vi "Handle Command.vi"(8 "error in (no error)":errorcluster, 9 "Data":variant, 10 "Command":string, 11 "Instrument.Lockin":refnum<class "Instrument.Lockin.lvclass">) -> (0 "error out":errorcluster, 1 "Processed Data":variant, 2 "Command":string, 3 "Instrument.Lockin out":refnum<class "Instrument.Lockin.lvclass">)   [LabVIEW 2019, in "Instrument.Lockin.lvlib" / "Instrument.Lockin.lvclass"]
uses:
  Instrument.Lockin.lvclass
  Typedefs/API/Lockin.Commands--Enum.ctl
  f7b28b50-f868-4d06-8d90-790d331e6843.vi
  Instrument.DAQ/Instrument.DAQ.lvclass
  Instrument.DAQ/Typedefs/AO.Channel.Function--Enum.ctl
  Instrument.DAQ/Typedefs/AO.Channel--Cluster.ctl
  06f5bff1-b823-416c-a758-fc672ecfcc99.vi
  Typedefs/API/Lockin.setAO_Amp--cluster.ctl
  029a7bc4-99e9-4f65-b437-c26585c9cd40.vi
  95117756-58c8-4cf5-b4a1-eea4f9571e2f.vi
  d527b0ad-2cbe-40d7-81d2-49d8d0078832.vi
  c6561379-f98d-4793-93aa-fc4f7b6fa2da.vi
  Typedefs/API/Lockin.setAO_DC--cluster.ctl
  Typedefs/API/Lockin.setAO_f--cluster.ctl
  Typedefs/API/Lockin.setAO_phi--cluster.ctl
  Typedefs/API/Lockin.setAO_function--cluster.ctl
  2465c698-e437-4a4f-8860-a626a4e5f6de.vi
  3b890341-4124-4342-9d75-403cba162ea7.vi
  efd52b93-d691-4a9b-b54f-f4c6778ec2a4.vi
  1b48001d-6f4c-40ce-9883-2cfdfc5b0066.vi
  451a16e7-7f0f-4872-98b2-f896a68061ac.vi
  Instrument.DAQ/Typedefs/REF.Channel--Cluster.ctl
  Typedefs/REF Parameter--Enum.ctl
  Typedefs/API/Lockin.setREF_f--cluster.ctl
  Typedefs/API/Lockin.setREF_phi--cluster.ctl
  Typedefs/API/Lockin.setREF_TC--cluster.ctl
  Typedefs/API/Lockin.setREF_RollOff--cluster.ctl
  Instrument.DAQ/Typedefs/State--enum.ctl
  afc408c1-4a47-494c-817e-7b9f9bb33729.vi
  Instrument.DAQ/Typedefs/Sweep.Pattern--Enum.ctl
  Instrument.DAQ/Typedefs/Sweep.Channel--Cluster.ctl
  Instrument.DAQ/Typedefs/Sweep.Configuration--Cluster.ctl
  ce862ac6-3818-4682-989c-38fcf43d7c0a.vi
  06811b67-d74b-4972-af3b-9250fa170671.vi
  Instrument.DAQ/Typedefs/DAQ.Sampling.Sampling--Cluster.ctl
  2eef0b96-7480-46b2-a416-598848f5f946.vi
  b666889e-e9d3-40fa-bff7-b740bef29075.vi
  Instrument.DAQ/Typedefs/DAQ.Config.AI.Coupling--enum.ctl
  Instrument.DAQ/Typedefs/DAQ.Config.AI.Range--enum.ctl
  Instrument.DAQ/Typedefs/DAQ.Config.AO.Range--enum.ctl
  Instrument.DAQ/Typedefs/DAQ.Configuration--Cluster.ctl
  4baefe16-dd55-4900-a34f-f85402a43af0.vi
  Instrument.DAQ/Typedefs/Sweep.Channel--Cluster--Array.ctl
  Instrument.DAQ/Typedefs/AO.Channel--Cluster--Array.ctl
  Instrument.DAQ/Typedefs/REF.Channel--Cluster--Array.ctl
  Instrument.DAQ/Typedefs/DAQ.Configuration--Cluster--Array.ctl
  df248ea2-cdbc-4a64-a66c-167358fcc18f.vi
  Instrument.DAQ/Typedefs/AI.Channel--Cluster.ctl
  Instrument.DAQ/Typedefs/AI.Channel--Cluster--Array.ctl
  Typedefs/Offset Mode--Enum.ctl
  Instrument.DAQ/Typedefs/Configuration.Prefilter--Cluster.ctl
  Typedefs/API/Lockin.Commands.Local--Enum.ctl
  Instrument.DAQ/Typedefs/Configuration.LinkFrequencies--Cluster.ctl
  Instrument.DAQ/Typedefs/Configuration.AmplitudeLimit--Cluster.ctl
  Instrument.DAQ/Typedefs/Simulation Mode--enum.ctl
  Instrument.DAQ/Typedefs/Channel.Gain--Cluster.ctl
  Instrument.DAQ/Typedefs/PrivateEvents--DAQ.setCalibration.ctl
  f4b2f717-a3e3-4701-aa1a-36f1ad587562.vi
  cb03029c-6dea-422e-9ff0-c01ba24202a7.vi
  ea7ae40a-427f-4df9-8330-54c2df2a5be0.vi
  d5077292-e533-4b52-a4d7-ebb5f6280e78.vi
  be7fa38f-04e0-4644-9c08-a6c1d8484273.vi
  228c5f99-5a8a-4ac9-8c3f-6c80f04cbb43.vi
  847e6f07-fde4-45b3-9907-c341240c9864.vi
  bf5afc16-6b2f-47bd-9035-54b404507785.vi
  Instrument.DAQ/Typedefs/PrivateEvents--DAQ.showUI.ctl
  Typedefs/API/Lockin.setState--cluster.ctl
  0f1e83ab-c55c-46b9-bca3-9d617c6a026d.vi
  Typedefs/API/Lockin.setSweep_Time--cluster.ctl
  c46d61d8-ad78-4a4f-bd83-bba7d42c3393.vi
  Typedefs/API/Lockin.setSweep_Table--cluster.ctl
  <userlib>/LevyLab/Instrument Framework/Instrument Types/Lockin/Instrument.LockinAPI.lvclass
  a7ccf487-04bf-437f-bc58-012293c091eb.vi
  Typedefs/API/Lockin.setLogMode--cluster.ctl
  7fa0c9c7-d96f-42eb-b083-8fec20da1e25.vi
  <userlib>/LevyLab/Instrument Framework/Instrument Types/Lockin/Typedefs/LockinAPI.SweepData--Cluster.ctl
  <userlib>/LevyLab/Instrument Framework/Instrument Types/Lockin/Typedefs/LockinAPI.Sampling.Sampling--Cluster.ctl
  <userlib>/LevyLab/Instrument Framework/Instrument Types/Lockin/Typedefs/LockinAPI.getState.states--enum.ctl
  29174cef-b5b4-4b3d-8dd9-d067235044c7.vi
  Instrument.DAQ/Typedefs/Configuration.DCLimit--Cluster.ctl
  Instrument.DAQ/Typedefs/DAQ.TerminalConfiguration--ring.ctl
  0557ee3d-f7cd-4618-85ce-94304b7e905c.vi
  Instrument.DAQ/Typedefs/Configuration.DutyCycle--Cluster.ctl
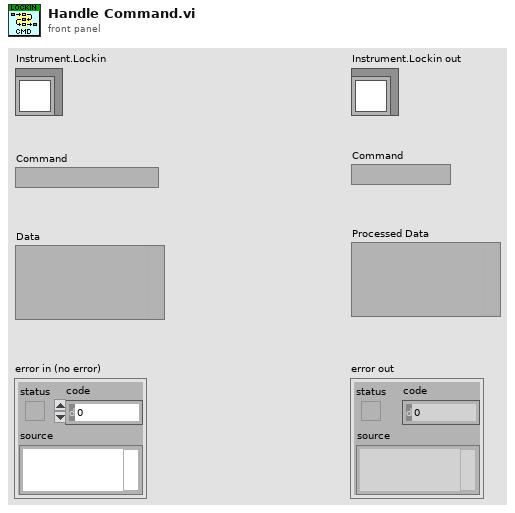
[diagram p1: front panel]
types:
  T1 = typedef "Instrument.Lockin.lvlib/Instrument.Lockin.lvclass/Lockin.Commands.Local--Enum.ctl" = enum16{"autoConfigureDAQ", "setSimulationMode", "zeroPhase", "setCalibration", "setPreFilter", "setFrequencyLink", "setAmplitudeLimit", "setDCLimit", "setDutyCycle", "setSamplingFsOutput", "setData_State", "setData_DAQ", "setData_Sampling", "setData_Waveforms", "setData_Results", "setData_SweepWaveforms", "setData_AIChannels", "setData_AOChannels", "setData_REFChannels", "setData_InputGain", "setData_OutputGain", "showUI", "setAI", "setOffset", "setOffsetMode"}
  T2 = typedef "Instrument.Lockin.lvlib/Instrument.Lockin.lvclass/Lockin.Commands--Enum.ctl" = enum16{"setAO", "setAO_Amplitude", "setAO_DC", "setAO_Frequency", "setAO_Phase", "setAO_Function", "setREF", "setREF_Frequency", "setREF_Phase", "setREF_TC", "setREF_Roll-Off", "setDAQ", "setSampling", "setState", "getState", "getAO", "getAI", "getResults", "getSampling", "getAOconfig", "getREFconfig", "setInputGain", "setOutputGain", "getInputGain", "getOutputGain", "setSweep", "setSweep_Time", "setSweep_Table", "getStatus", "getSweepResults", "getSweepWaveforms", "logConfiguration", "startLogging", "stopLogging"}
  T3 = typedef "Instrument.LockinAPI.lvclass/LockinAPI.Sampling.Sampling--Cluster.ctl" = cluster{"Fs":dbl, "#s":i32}
  T4 = typedef "Instrument.LockinAPI.lvclass/LockinAPI.getState.states--enum.ctl" = enum16{"idle", "created", "started", "stopped", "sweeping"}
  T5 = typedef "Instrument.LockinAPI.lvclass/LockinAPI.SweepData--Cluster.ctl" = cluster{"AO":waveform(dbl)[], "AI":waveform(dbl)[], "X":waveform(dbl)[], "Y":waveform(dbl)[]}
  T6 = cluster{"Time Stamp":timestamp, "Results (Dictionary)":cluster{"key":string, "value":dbl}[]}
  T7 = typedef "Instrument.Lockin.lvlib/Instrument.Lockin.lvclass/Lockin.setState--cluster.ctl" = cluster{"State":T8}
  T8 = typedef "Instrument.Lockin.lvlib/Instrument.DAQ.lvclass/State--enum.ctl" = enum16{"start", "stop", "reset", "start sweep", "stop sweep"}
  T9 = typedef "Instrument.Lockin.lvlib/Instrument.Lockin.lvclass/Lockin.setLogMode--cluster.ctl" = cluster{"interval":u32}
  T10 = enum16{"Amplitude", "DC", "Frequency", "Phase", "Function"}
  T11 = typedef "Instrument.Lockin.lvlib/Instrument.Lockin.lvclass/Lockin.setAO_Amp--cluster.ctl" = cluster{"Channel":i32, "Amplitude":dbl}
  T12 = typedef "Instrument.Lockin.lvlib/Instrument.Lockin.lvclass/Lockin.setAO_DC--cluster.ctl" = cluster{"Channel":i32, "DC":dbl}
  T13 = typedef "Instrument.Lockin.lvlib/Instrument.Lockin.lvclass/Lockin.setAO_f--cluster.ctl" = cluster{"Channel":i32, "Frequency":dbl}
  T14 = typedef "Instrument.Lockin.lvlib/Instrument.Lockin.lvclass/Lockin.setAO_phi--cluster.ctl" = cluster{"Channel":i32, "Phase":dbl}
  T15 = typedef "Instrument.Lockin.lvlib/Instrument.Lockin.lvclass/Lockin.setAO_function--cluster.ctl" = cluster{"Channel":i32, "Function":T16}
  T16 = typedef "Instrument.Lockin.lvlib/Instrument.DAQ.lvclass/AO.Channel.Function--Enum.ctl" = enum16{"sine", "square", "triangle", "saw"}
  T17 = typedef "Instrument.Lockin.lvlib/Instrument.DAQ.lvclass/AO.Channel--Cluster--Array.ctl" = T18[]
  T18 = typedef "Instrument.Lockin.lvlib/Instrument.DAQ.lvclass/AO.Channel--Cluster.ctl" = cluster{"Enable?":bool, "Channel":i32, "Amplitude":dbl, "Offset":dbl, "Frequency":dbl, "Phase":dbl, "Function":T16, "Sweeping?":bool, "Limit AC":bool, "Limit DC?":bool, "Duty Cycle":bool}
  T19 = typedef "Instrument.Lockin.lvlib/Instrument.Lockin.lvclass/Lockin.setREF_f--cluster.ctl" = cluster{"Channel":i32, "Frequency":dbl}
  T20 = typedef "Instrument.Lockin.lvlib/Instrument.Lockin.lvclass/REF Parameter--Enum.ctl" = enum16{"Frequency", "Phase", "Time Constant", "RollOff"}
  T21 = typedef "Instrument.Lockin.lvlib/Instrument.Lockin.lvclass/Lockin.setREF_phi--cluster.ctl" = cluster{"Channel":i32, "Phase":dbl}
  T22 = typedef "Instrument.Lockin.lvlib/Instrument.Lockin.lvclass/Lockin.setREF_TC--cluster.ctl" = cluster{"Channel":i32, "TC":dbl}
  T23 = typedef "Instrument.Lockin.lvlib/Instrument.Lockin.lvclass/Lockin.setREF_RollOff--cluster.ctl" = cluster{"Channel":i32, "Roll-Off":i32}
  T24 = typedef "Instrument.Lockin.lvlib/Instrument.DAQ.lvclass/REF.Channel--Cluster--Array.ctl" = T25[]
  T25 = typedef "Instrument.Lockin.lvlib/Instrument.DAQ.lvclass/REF.Channel--Cluster.ctl" = cluster{"Enable?":bool, "Channel":i32, "Frequency":dbl, "Phase":dbl, "TC":dbl, "Roll-Off":i32}
  T26 = typedef "Instrument.Lockin.lvlib/Instrument.Lockin.lvclass/Lockin.setSweep_Time--cluster.ctl" = cluster{"SweepTime":dbl}
  T27 = typedef "Instrument.Lockin.lvlib/Instrument.Lockin.lvclass/Lockin.setSweep_Table--cluster.ctl" = cluster{"Channel":i32, "Table":dbl[]}
  T28 = typedef "Instrument.Lockin.lvlib/Instrument.DAQ.lvclass/DAQ.Sampling.Sampling--Cluster.ctl" = cluster{"Fs":dbl, "#s":i32}
  T29 = typedef "Instrument.Lockin.lvlib/Instrument.DAQ.lvclass/Channel.Gain--Cluster.ctl" = cluster{"Channel":string, "Gain":dbl}
  T30 = typedef "Instrument.Lockin.lvlib/Instrument.DAQ.lvclass/DAQ.Configuration--Cluster--Array.ctl" = T31[]
  T31 = typedef "Instrument.Lockin.lvlib/Instrument.DAQ.lvclass/DAQ.Configuration--Cluster.ctl" = cluster{"Device":string, "Lockin.AO":string, "AO.Ch":string, "AO.Range":T32, "AO terminal config":T33, "Lockin.AI":string, "AI.Ch":string, "AI.Range":T34, "AI.Coupling":T35, "AI terminal config":T33}
  T32 = typedef "Instrument.Lockin.lvlib/Instrument.DAQ.lvclass/DAQ.Config.AO.Range--enum.ctl" = enum16{"±0.1", "±1.0", "±3.5", "±10.0", ""}
  T33 = typedef "Instrument.Lockin.lvlib/Instrument.DAQ.lvclass/DAQ.TerminalConfiguration--ring.ctl" = i32
  T34 = typedef "Instrument.Lockin.lvlib/Instrument.DAQ.lvclass/DAQ.Config.AI.Range--enum.ctl" = enum16{"±0.316", "±1.00", "±3.16", "±10.0", "±31.6", "±42.4", ""}
  T35 = typedef "Instrument.Lockin.lvlib/Instrument.DAQ.lvclass/DAQ.Config.AI.Coupling--enum.ctl" = u16
  T36 = typedef "Instrument.Lockin.lvlib/Instrument.DAQ.lvclass/PrivateEvents--DAQ.showUI.ctl" = bool
  T37 = typedef "Instrument.Lockin.lvlib/Instrument.DAQ.lvclass/AI.Channel--Cluster--Array.ctl" = T38[]
  T38 = typedef "Instrument.Lockin.lvlib/Instrument.DAQ.lvclass/AI.Channel--Cluster.ctl" = cluster{"Enable?":bool, "Channel":i32, "References":u16[], "reference index":i32}
  T39 = typedef "Instrument.Lockin.lvlib/Instrument.DAQ.lvclass/Simulation Mode--enum.ctl" = enum16{"AI = HW simulated", "AI = noise*AO", "AI = waveguide"}
  T40 = typedef "Instrument.Lockin.lvlib/Instrument.Lockin.lvclass/Offset Mode--Enum.ctl" = enum16{"Measure", "Remove"}
  T41 = typedef "Instrument.Lockin.lvlib/Instrument.DAQ.lvclass/PrivateEvents--DAQ.setCalibration.ctl" = enum16{"Check", "Calibrate"}
  T42 = typedef "Instrument.Lockin.lvlib/Instrument.DAQ.lvclass/Configuration.Prefilter--Cluster.ctl" = cluster{"60 Hz":bool, "Low Pass":bool, "Low Pass Cutoff (Hz)":dbl}
  T43 = typedef "Instrument.Lockin.lvlib/Instrument.DAQ.lvclass/Configuration.LinkFrequencies--Cluster.ctl" = cluster{"Link?":bool, "Frequency (Hz)":dbl}
  T44 = typedef "Instrument.Lockin.lvlib/Instrument.DAQ.lvclass/Configuration.DCLimit--Cluster.ctl" = cluster{"Limit (V)":dbl}
  T45 = typedef "Instrument.Lockin.lvlib/Instrument.DAQ.lvclass/Configuration.DutyCycle--Cluster.ctl" = cluster{"Option?":bool, "Duty Cycle (%)":dbl}
  T46 = typedef "Instrument.Lockin.lvlib/Instrument.DAQ.lvclass/Status--enum.ctl" = enum16{"idle", "created", "started", "stopped", "sweeping"}
  T47 = typedef "Instrument.Lockin.lvlib/Instrument.DAQ.lvclass/Channel.Gain--Cluster--Array.ctl" = T29[]
  T48 = typedef "Instrument.Lockin.lvlib/Instrument.DAQ.lvclass/Results--Cluster.ctl" = cluster{"Time Stamp":timestamp, "Results (Dictionary)":cluster{"key":string, "value":dbl[]}[]}
  T49 = typedef "Instrument.Lockin.lvlib/Instrument.DAQ.lvclass/Sweep.Configuration--Cluster.ctl" = cluster{"sweepTime":dbl, "initialWaitTime":dbl, "returnToStart":bool, "sweepChannels":T50}
  T50 = typedef "Instrument.Lockin.lvlib/Instrument.DAQ.lvclass/Sweep.Channel--Cluster--Array.ctl" = T51[]
  T51 = typedef "Instrument.Lockin.lvlib/Instrument.DAQ.lvclass/Sweep.Channel--Cluster.ctl" = cluster{"Enable?":bool, "Channel":u16, "Start":dbl, "End":dbl, "Pattern":T52, "Table":dbl[]}
  T52 = typedef "Instrument.Lockin.lvlib/Instrument.DAQ.lvclass/Sweep.Pattern--Enum.ctl" = enum16{"Ramp /", "Ramp /\\", "Smooth Ramp _/", "Smooth Ramp _/\\_", "Table"}
  T53 = typedef "Instrument.Lockin.lvlib/Instrument.DAQ.lvclass/DAQ.Sampling--Cluster.ctl" = cluster{"Sampling":T28, "Fs_Out":dbl}
  T54 = typedef "Instrument.Lockin.lvlib/Instrument.DAQ.lvclass/DAQ.Config.AO--Cluster--Array.ctl" = cluster{"Channels":tag, "Range":T32, "terminal configuration":T33, "Type":T55}[]
  T55 = typedef "Instrument.Lockin.lvlib/Instrument.DAQ.lvclass/DAQ.Type--enum.ctl" = enum16{"None", "USB-4431", "PXI-446x"}
  T56 = typedef "Instrument.Lockin.lvlib/Instrument.DAQ.lvclass/DAQ.Config.AI--Cluster--Array.ctl" = cluster{"Channels":tag, "Coupling":T35, "Range":T34, "terminal configuration":T33, "Type":T55}[]
  T57 = typedef "Instrument.Lockin.lvlib/Instrument.DAQ.lvclass/PublicEvents--DAQ.getWaveforms.ctl" = cluster{"AO":waveform(dbl)[], "AI":waveform(dbl)[], "REF_X":waveform(dbl)[], "REF_Y":waveform(dbl)[], "X":waveform(dbl)[], "Y":waveform(dbl)[]}
  T58 = typedef "Instrument.Lockin.lvlib/Instrument.DAQ.lvclass/PublicEvents--DAQ.getSweepWaveforms.ctl" = cluster{"AO":waveform(dbl)[], "AI":waveform(dbl)[], "X":waveform(dbl)[], "Y":waveform(dbl)[]}
  T59 = typedef "Instrument.Lockin.lvlib/Instrument.DAQ.lvclass/Configuration.AmplitudeLimit--Cluster.ctl" = cluster{"Limit (V)":dbl}
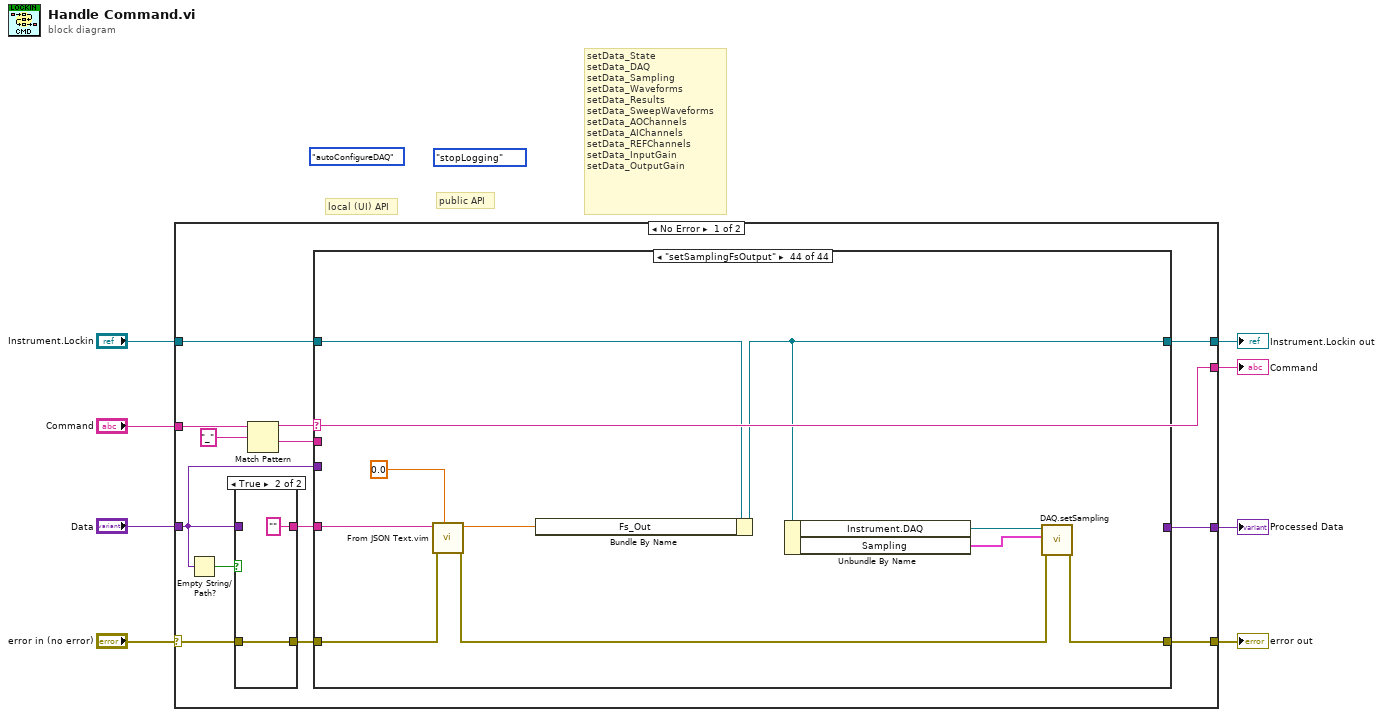
[diagram p0: block diagram]
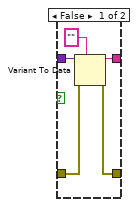
[diagram p2: hidden frame]
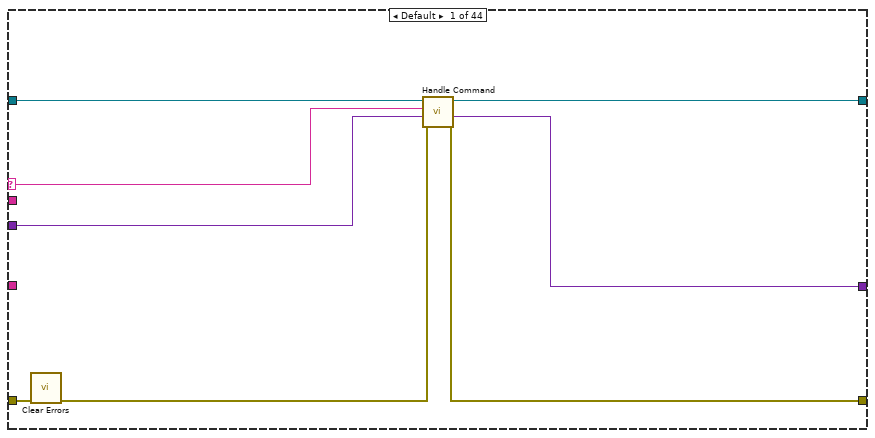
[diagram p3: hidden frame]
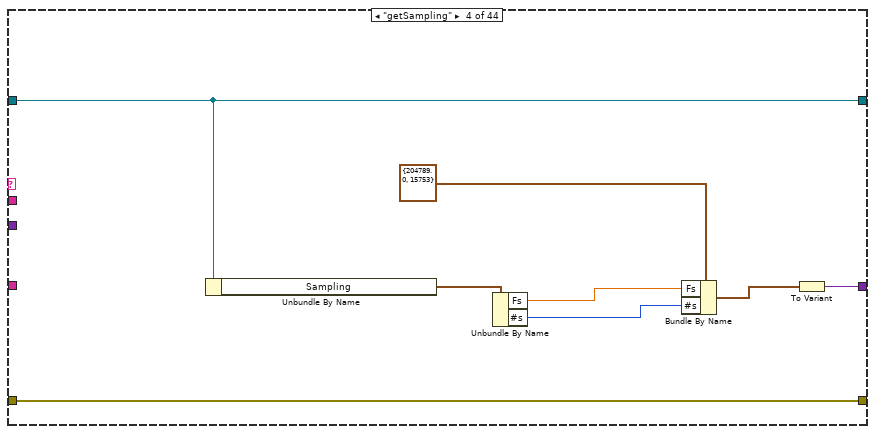
[diagram p6: hidden frame]
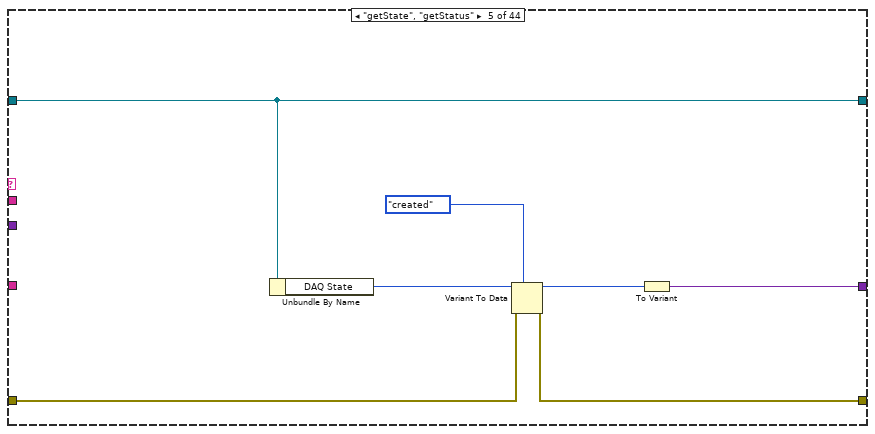
[diagram p7: hidden frame]
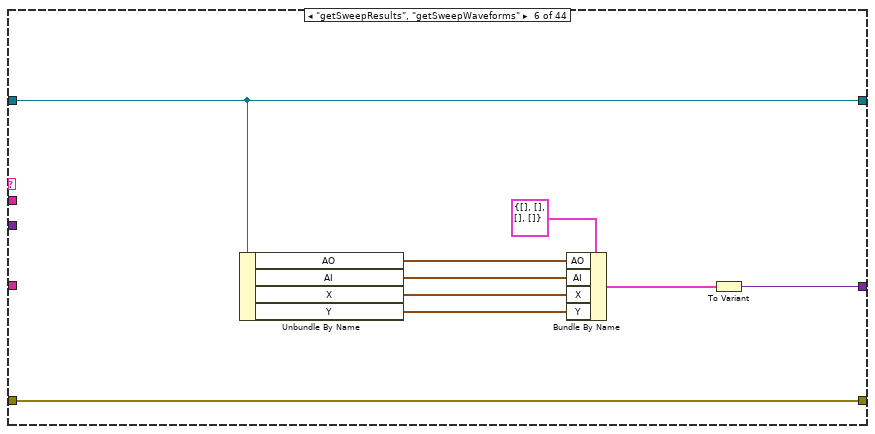
[diagram p8: hidden frame]
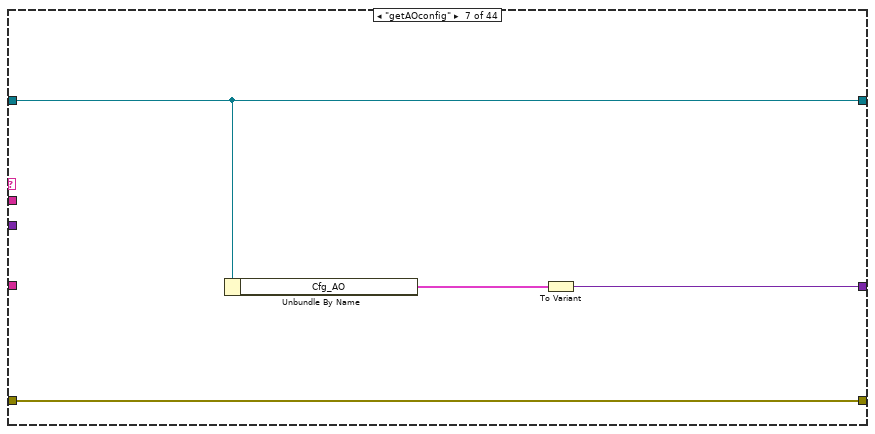
[diagram p9: hidden frame]
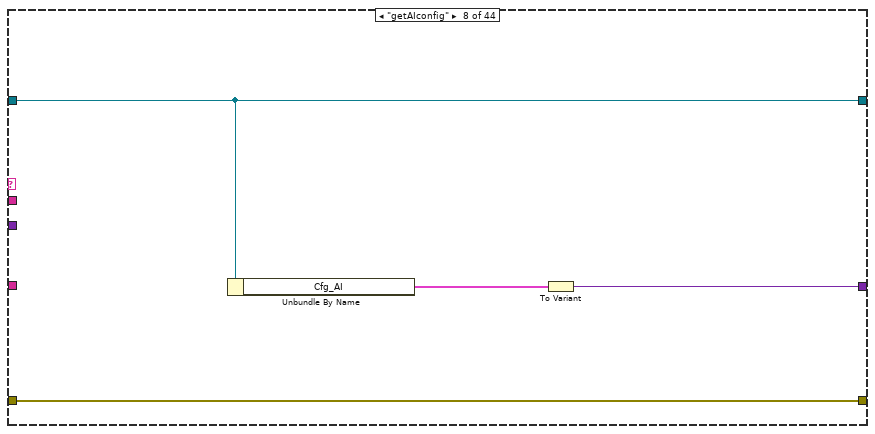
[diagram p10: hidden frame]
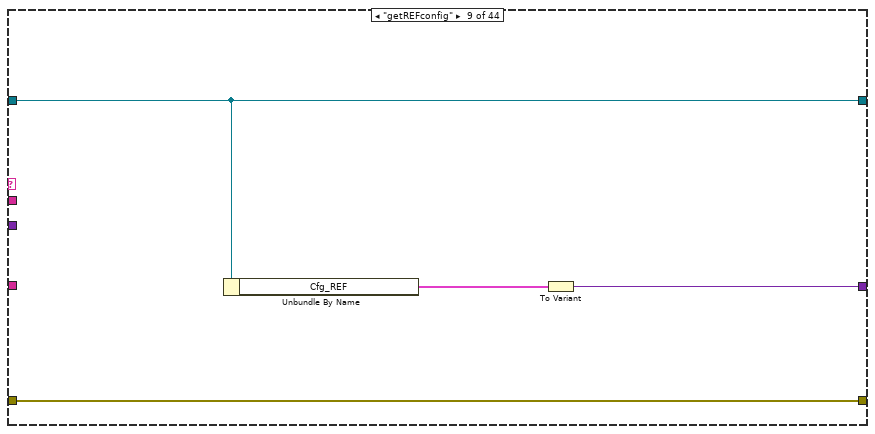
[diagram p11: hidden frame]
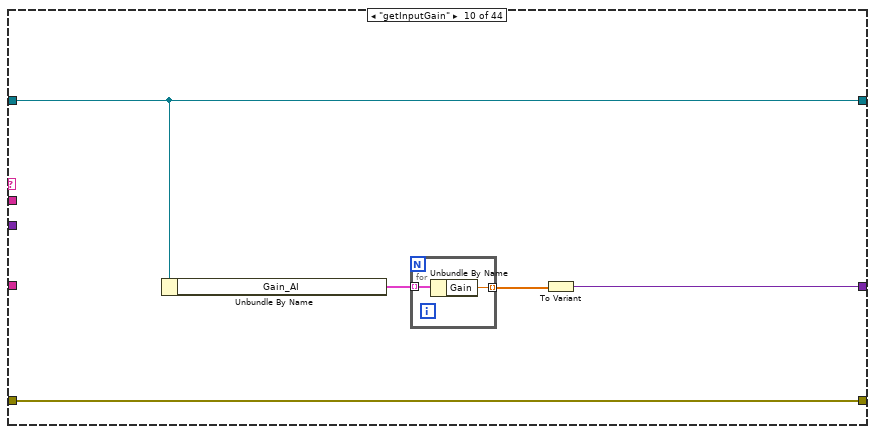
[diagram p12: hidden frame]
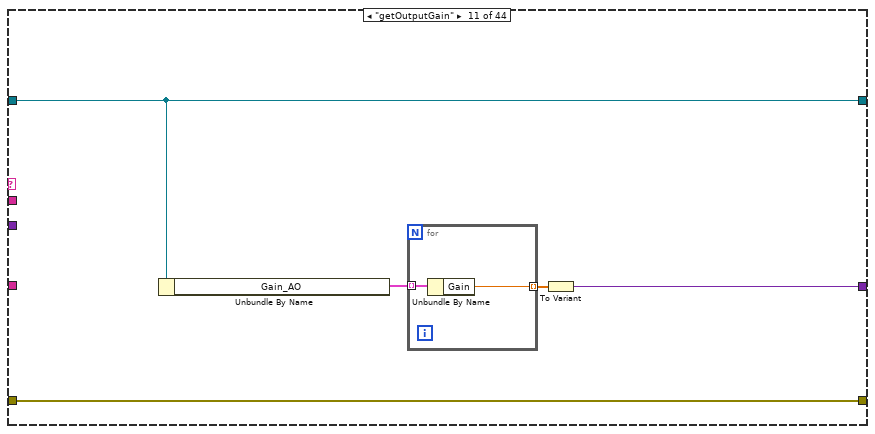
[diagram p13: hidden frame]
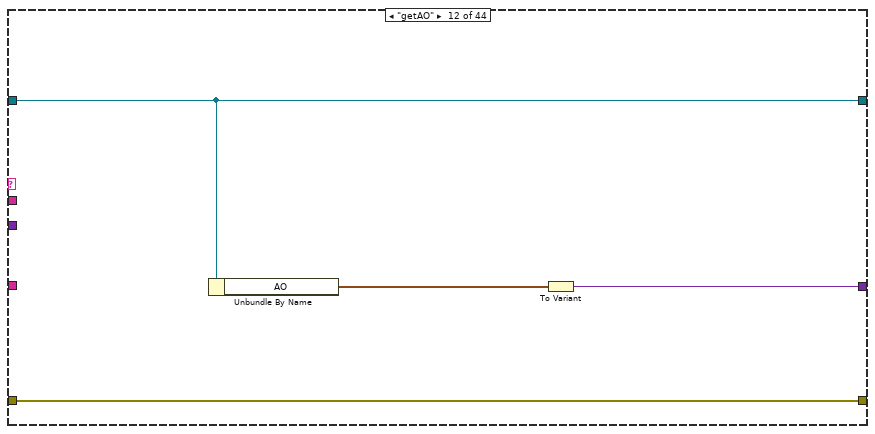
[diagram p14: hidden frame]
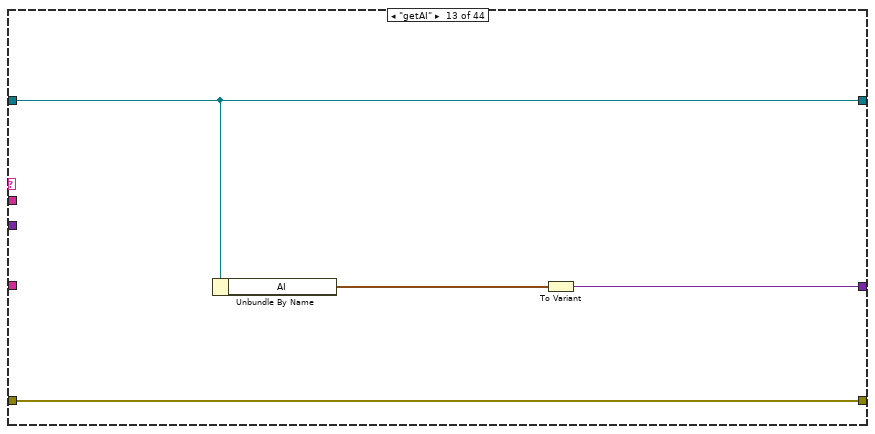
[diagram p15: hidden frame]
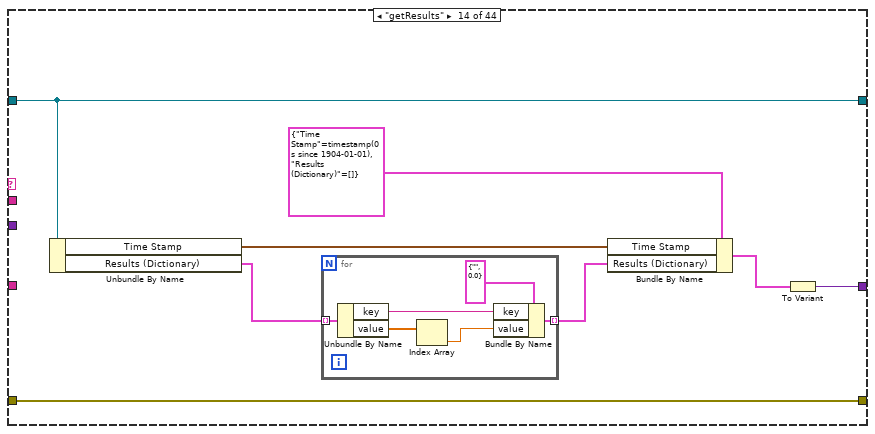
[diagram p16: hidden frame]
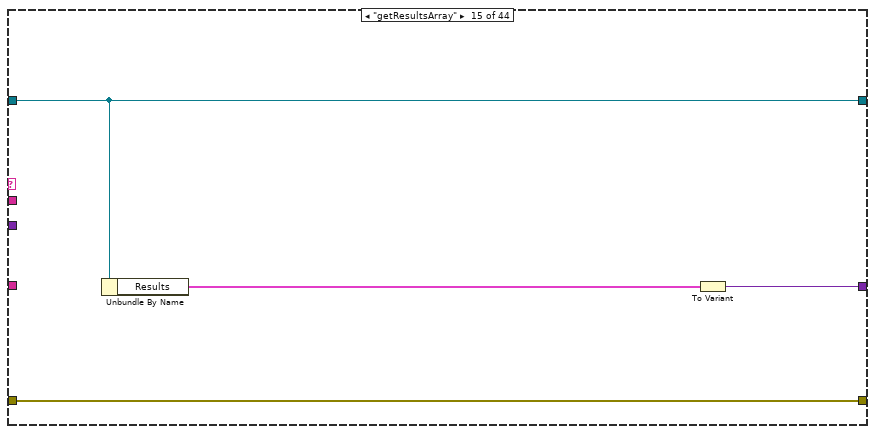
[diagram p17: hidden frame]
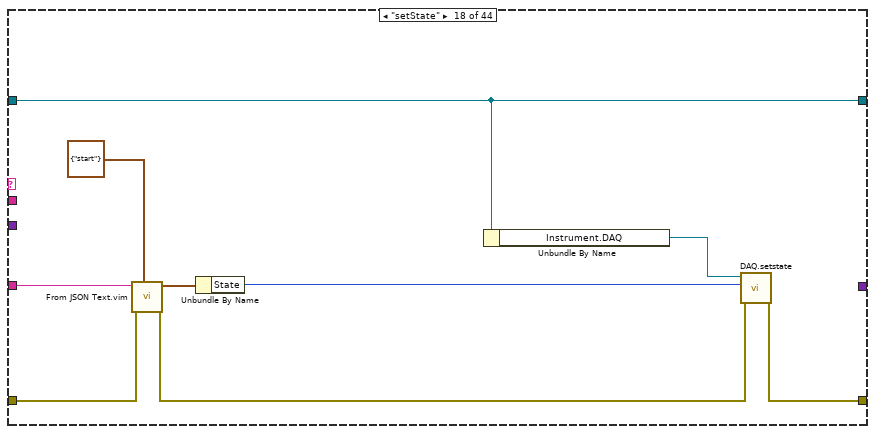
[diagram p20: hidden frame]
diagram:
  (unwired) Lockin.Commands.Local--Enum."autoConfigureDAQ" ("Enum")
  (unwired) Lockin.Commands--Enum."stopLogging" ("Enum")
  # "setData_State\nsetData_DAQ\nsetData_Sampling\nsetData_Waveforms\nsetData_Results\nsetData_SweepWaveforms\nsetData_AOChannels\nsetData_AIChannels\nsetData_REFChannels\nsetData_InputGain\nsetData_OutputGain"
  # "local (UI) API"
  # "public API"
  n1 = case shown="No Error" "error in (no error)" {
    selector: "error in (no error)" -> [w17 w639]
    tunnel: [w18 w639] -> w7
    tunnel: [w20 w638] -> w6
    tunnel: "Instrument.Lockin" -> [w21 w638]
    tunnel: "Command" -> [w12 w637]
    tunnel: [w19 variant] -> w5
    tunnel: "Data" -> [w9 _]
    tunnel: [w11 w637] -> w3
    frame No Error {
      n2 = Empty String/Path?(string/path=w9) -> (empty?=w10:bool)
      n3 = case shown="True" w10 {
        tunnel: w17 -> [w26 w27]
        tunnel: [w24 ""] -> w16
        tunnel: [w23 w27] -> w13
        tunnel: w9 -> [w22 _]
        frame False {
          n4 = Variant To Data(error in=w26, type="", Variant=w22) -> (data=w24:string, error out=w23:errorcluster)
        }
        frame True {
        }
      }
      n5 = Match Pattern(string=w12, regular expression="_") -> (before substring=w11:string, after substring=w14:string)  [unwired: 1 in, 2 out]
      n6 = case shown="\"setSamplingFsOutput\"" w11 {
        selector: w11 -> [w31 _ _ _ _ _ _ _ _ _ _ _ _ _ _ _ _ _ _ _ _ _ _ _ _ _ _ _ _ _ _ _ _ _ _ _ _ _ _ _ _ _ _ _]
        tunnel: w21 -> [w36 w38 w40 w46 w54 w62 w65 w69 w73 w79 w86 w91 w95 w104 w114 w118 w120 w124 w133 w140 w144 w149 w223 w286 w318 w331 w349 w368 w385 w396 w398 w412 w420 w534 w547 w557 w567 w575 w582 w594 w604 w614 w624 w635]
        tunnel: [w34 w38 w40 w46 w54 w62 w65 w69 w73 w79 w86 w91 w95 w104 w114 w118 w120 w124 w133 w140 w144 w147 w218 w290 w317 w332 w350 w369 w384 w396 w398 w406 w416 w534 w546 w557 w567 w575 w583 w595 w605 w615 w625 w632] -> w20
        tunnel: [w35 _ _ w48 w55 w64 w67 w71 w75 w81 w88 w94 w98 w106 w116 _ _ _ _ _ _ _ _ _ _ _ _ _ _ _ _ _ _ _ _ w548 _ _ _ _ _ _ _ _] -> w19
        tunnel: w16 -> [_ _ _ _ _ _ _ _ _ _ _ _ _ _ _ _ _ w129 w137 _ _ w153 w226 w294 w324 w337 w355 w373 w394 _ w404 w414 w418 _ w541 w554 _ w572 w579 w590 w600 w613 w623 w629]
        tunnel: [w32 w37 w39 w47 w50 w63 w66 w70 w74 w80 w87 w93 w97 w105 w115 w117 w119 w125 w130 w139 w143 w150 w219 w291 w320 w333 w351 w370 w389 w395 w399 w408 w415 w536 w542 w555 w565 w573 w584 w591 w601 w607 w616 w631] -> w18
        tunnel: w14 -> [_ _ _ _ _ _ _ _ _ _ _ _ _ _ _ _ _ _ _ _ _ w148 w224 w287 _ _ _ _ _ _ _ _ w419 _ _ _ _ _ _ _ _ _ _ _]
        tunnel: w13 -> [w33 w37 w39 w47 w49 w63 w66 w70 w74 w80 w87 w93 w97 w105 w115 w117 w119 w128 w136 w138 w141 w152 w225 w293 w322 w336 w354 w372 w393 w395 w401 w413 w417 w535 w540 w551 w566 w568 w577 w588 w597 w611 w621 w628]
        tunnel: w9 -> [w30 _ _ _ _ _ _ _ _ _ _ _ _ _ _ _ _ _ _ _ _ _ _ _ _ _ _ _ _ _ _ _ _ _ _ _ _ _ _ _ _ _ _ _]
        frame Default {
          n7 = call <vilib>:"Clear Errors.vi"("error in (no error)"=w33) -> ("error out"=w29:errorcluster)  [unwired: 5 in, 1 out]
          n8 = call-parent "Handle Command.vi"("error in (no error)"=w29, "params in"=w30, "command"=w31, "Instrument in"=w36) -> ("error out"=w32:errorcluster, "processed data"=w35:variant, "Instrument out"=w34:refnum<class "Instrument.Lockin.lvclass">)  [unwired: 4 in, 1 out]
        }
        frame "----------PUBLIC API----------" {
        }
        frame "----------GET METHODS----------" {
        }
        frame "getSampling" {
          n9 = Unbundle By Name(w46) -> ("Sampling"=w44:T28)
          n10 = Unbundle By Name(w44) -> ("Fs"=w43:dbl, "#s"=w42:i32)
          n11 = Bundle By Name(cluster=T3 {"Fs"=204789.0, "#s"=15753} ("sampling"), "Fs"=w43, "#s"=w42) -> (w41:T3)
          n12 = To Variant(anything=w41) -> (Variant=w48:variant)
        }
        frame "getState", "getStatus" {
          n13 = Unbundle By Name(w54) -> ("DAQ State"=w52:T46)
          n14 = Variant To Data(error in=w49, type=LockinAPI.getState.states--enum."created" ("getState.states"), Variant=w52) -> (data=w51:T4, error out=w50:errorcluster)
          n15 = To Variant(anything=w51) -> (Variant=w55:variant)
        }
        frame "getSweepResults", "getSweepWaveforms" {
          n16 = Unbundle By Name(w62) -> ("AO"=w60:waveform(dbl)[], "AI"=w59:waveform(dbl)[], "X"=w58:waveform(dbl)[], "Y"=w57:waveform(dbl)[])
          n17 = Bundle By Name(cluster=T5 {"AO"=[], "AI"=[], "X"=[], "Y"=[]} ("sweepData"), "AO"=w60, "AI"=w59, "X"=w58, "Y"=w57) -> (w56:T5)
          n18 = To Variant(anything=w56) -> (Variant=w64:variant)
        }
        frame "getAOconfig" {
          n19 = Unbundle By Name(w65) -> ("Cfg_AO"=w68:T17)
          n20 = To Variant(anything=w68) -> (Variant=w67:variant)
        }
        frame "getAIconfig" {
          n21 = Unbundle By Name(w69) -> ("Cfg_AI"=w72:T37)
          n22 = To Variant(anything=w72) -> (Variant=w71:variant)
        }
        frame "getREFconfig" {
          n23 = Unbundle By Name(w73) -> ("Cfg_REF"=w76:T24)
          n24 = To Variant(anything=w76) -> (Variant=w75:variant)
        }
        frame "getInputGain" {
          n25 = Unbundle By Name(w79) -> ("Gain_AI"=w78:T47)
          n26 = for {
            tunnel: w78 -> [w83] mode=indexing
            tunnel: [w82] -> w77 mode=indexing
            n27 = Unbundle By Name(w83) -> ("Gain"=w82:dbl)
          }
          n28 = To Variant(anything=w77) -> (Variant=w81:variant)
        }
        frame "getOutputGain" {
          n29 = Unbundle By Name(w86) -> ("Gain_AO"=w85:T47)
          n30 = for {
            tunnel: w85 -> [w90] mode=indexing
            tunnel: [w89] -> w84 mode=indexing
            n31 = Unbundle By Name(w90) -> ("Gain"=w89:dbl)
          }
          n32 = To Variant(anything=w84) -> (Variant=w88:variant)
        }
        frame "getAO" {
          n33 = Unbundle By Name(w91) -> ("AO"=w92:waveform(dbl)[])
          n34 = To Variant(anything=w92) -> (Variant=w94:variant)
        }
        frame "getAI" {
          n35 = Unbundle By Name(w95) -> ("AI"=w96:waveform(dbl)[])
          n36 = To Variant(anything=w96) -> (Variant=w98:variant)
        }
        frame "getResults" {
          n37 = Unbundle By Name(w104) -> ("Time Stamp"=w101:timestamp, "Results (Dictionary)"=w100:cluster{"key":string, "value":dbl[]}[])
          n38 = for {
            tunnel: w100 -> [w111] mode=indexing
            tunnel: [w107] -> w102 mode=indexing
            n39 = Unbundle By Name(w111) -> ("key"=w108:string, "value"=w112:dbl[])
            n40 = Index Array(array=w112) -> (element=w109:dbl)  [unwired: 1 in]
            n41 = Bundle By Name(cluster=cluster{"key":string, "value":dbl} {"key"="", "value"=0.0} ("key-value"), "key"=w108, "value"=w109) -> (w107:cluster{"key":string, "value":dbl})
          }
          n42 = Bundle By Name(cluster=T6 {"Time Stamp"=timestamp(0 s since 1904-01-01), "Results (Dictionary)"=[]} ("input cluster"), "Time Stamp"=w101, "Results (Dictionary)"=w102) -> (w99:T6)
          n43 = To Variant(anything=w99) -> (Variant=w106:variant)
        }
        frame "getResultsArray" {
          n44 = Unbundle By Name(w114) -> ("Results"=w113:T48)
          n45 = To Variant(anything=w113) -> (Variant=w116:variant)
        }
        frame "getAUX" {
        }
        frame "----------SET METHODS----------" {
        }
        frame "setState" {
          n46 = call "From JSON Text.vim"("Data Type and Default Value"=T7 {"State"=enum."start"} ("setState"), "error in (no error)"=w128, "JSON"=w129) -> ("error out"=w126:errorcluster, "Data out"=w122:T7)  [unwired: 7 in]
          n47 = Unbundle By Name(w122) -> ("State"=w121:T8)
          n48 = Unbundle By Name(w124) -> ("Instrument.DAQ"=w127:refnum<class "Instrument.DAQ.lvclass">)
          n49 = call "DAQ.setstate.vi"("error in (no error)"=w126, "setState"=w121, "Instrument.DAQ"=w127) -> ("error out"=w125:errorcluster)  [unwired: 7 in, 1 out]
        }
        frame "startLogging" {
          # "local event API does not need cluster"
          # "remote API store data in cluster"
          n50 = call "From JSON Text.vim"("Data Type and Default Value"=T9 {"interval"=1} ("setLogMode"), "error in (no error)"=w136, "JSON"=w137) -> ("error out"=w131:errorcluster, "Data out"=w135:T9)  [unwired: 7 in]
          n51 = Unbundle By Name(w135) -> ("interval"=w132:u32)
          n52 = call "Lockin.setLogMode.vi"("error in (no error)"=w131, "interval (ms)"=w132, "Instrument.Lockin"=w133) -> ("error out"=w130:errorcluster)  [unwired: 7 in, 1 out]
        }
        frame "logConfiguration" {
          # "local event API does not need cluster"
          # "remote API store data in cluster"
          n53 = call "Lockin.logConfiguration.vi"("error in (no error)"=w138, "Instrument.Lockin"=w140) -> ("error out"=w139:errorcluster)  [unwired: 8 in, 1 out]
        }
        frame "stopLogging" {
          # "local event API does not need cluster"
          n54 = call "Lockin.setLogMode.vi"("error in (no error)"=w141, "interval (ms)"=u32 0 ("interval"), "Instrument.Lockin"=w144) -> ("error out"=w143:errorcluster)  [unwired: 7 in, 1 out]
        }
        frame "setAO" {
          # "Lockin SMO: Set AO"
          # "Adjust Channels"
          n55 = case shown="\"\"" w148 {
            selector: w148 -> [w163 _]
            tunnel: w153 -> [w162 w215]
            tunnel: w152 -> [w161 w214]
            tunnel: [w156 w210] -> w146
            tunnel: w149 -> [w159 w213]
            tunnel: [w160 w212] -> w147
            frame Default {
              n56 = case shown="\"Phase\"" w163 {
                tunnel: w162 -> [w172 w181 w190 w199 w208]
                tunnel: w161 -> [w171 w180 w189 w198 w207]
                tunnel: [w170 w179 w188 w197 w206] -> w157
                tunnel: [T10."Amplitude" ("Parameter") T10."DC" ("Parameter") T10."Frequency" ("Parameter") T10."Phase" ("Parameter") T10."Function" ("Parameter")] -> w158
                tunnel: [w166 w176 w185 w194 w203] -> w155
                tunnel: [w164 w173 w182 w191 w200] -> w154
                frame "Amplitude", Default {
                  n57 = call "From JSON Text.vim"("Data Type and Default Value"=T11 {"Channel"=5, "Amplitude"=0.0} ("setAO_Amp"), "error in (no error)"=w171, "JSON"=w172) -> ("error out"=w170:errorcluster, "Data out"=w168:T11)  [unwired: 7 in]
                  n58 = Unbundle By Name(w168) -> ("Channel"=w166:i32, "Amplitude"=w165:dbl)
                  n59 = To Variant(anything=w165) -> (Variant=w164:variant)
                }
                frame "DC" {
                  n60 = call "From JSON Text.vim"("Data Type and Default Value"=T12 {"Channel"=5, "DC"=0.0} ("setAO_DC"), "error in (no error)"=w180, "JSON"=w181) -> ("error out"=w179:errorcluster, "Data out"=w178:T12)  [unwired: 7 in]
                  n61 = Unbundle By Name(w178) -> ("Channel"=w176:i32, "DC"=w175:dbl)
                  n62 = To Variant(anything=w175) -> (Variant=w173:variant)
                }
                frame "Frequency" {
                  n63 = call "From JSON Text.vim"("Data Type and Default Value"=T13 {"Channel"=5, "Frequency"=0.0} ("setAO_f"), "error in (no error)"=w189, "JSON"=w190) -> ("error out"=w188:errorcluster, "Data out"=w187:T13)  [unwired: 7 in]
                  n64 = Unbundle By Name(w187) -> ("Channel"=w185:i32, "Frequency"=w184:dbl)
                  n65 = To Variant(anything=w184) -> (Variant=w182:variant)
                }
                frame "Phase" {
                  n66 = call "From JSON Text.vim"("Data Type and Default Value"=T14 {"Channel"=5, "Phase"=0.0} ("setAO_phi"), "error in (no error)"=w198, "JSON"=w199) -> ("error out"=w197:errorcluster, "Data out"=w196:T14)  [unwired: 7 in]
                  n67 = Unbundle By Name(w196) -> ("Channel"=w194:i32, "Phase"=w193:dbl)
                  n68 = To Variant(anything=w193) -> (Variant=w191:variant)
                }
                frame "Function" {
                  n69 = call "From JSON Text.vim"("Data Type and Default Value"=T15 {"Channel"=5, "Function"=enum."sine"} ("setAO_function"), "error in (no error)"=w207, "JSON"=w208) -> ("error out"=w206:errorcluster, "Data out"=w205:T15)  [unwired: 7 in]
                  n70 = Unbundle By Name(w205) -> ("Channel"=w203:i32, "Function"=w202:T16)
                  n71 = To Variant(anything=w202) -> (Variant=w200:variant)
                }
              }
              n72 = call "Update AO Parameter.vi"("Parameter"=w158, "error in"=w157, "Value"=w154, "Channel"=w155, "Instrument.Lockin"=w159) -> ("error out"=w156:errorcluster, "Instrument.Lockin out"=w160:refnum<class "Instrument.Lockin.lvclass">)  [unwired: 5 in]
            }
            frame "" {
              n73 = call "From JSON Text.vim"("Data Type and Default Value"=T17 [] ("AO Channels"), "error in (no error)"=w214, "JSON"=w215) -> ("error out"=w210:errorcluster, "Data out"=w211:T17)  [unwired: 7 in]
              n74 = Bundle By Name(cluster=w213, "Cfg_AO"=w211) -> (w212:refnum<class "Instrument.Lockin.lvclass">)
            }
          }
          n75 = Unbundle By Name(w147) -> ("Instrument.DAQ"=w151:refnum<class "Instrument.DAQ.lvclass">, "Cfg_AO"=w145:T17)
          n76 = call "DAQ.setAO.vi"("error in (no error)"=w146, "AO Channels"=w145, "Instrument.DAQ"=w151) -> ("error out"=w150:errorcluster)  [unwired: 7 in, 1 out]
        }
        frame "setREF" {
          # "Lockin SMO: Set REF"
          # "Adjust Channels"
          n77 = case shown="Default" w224 {
            selector: w224 -> [w240 _]
            tunnel: w226 -> [w239 w283]
            tunnel: w225 -> [w238 w282]
            tunnel: [w235 w278] -> w217
            tunnel: w223 -> [w237 w281]
            tunnel: [w236 w280] -> w218
            frame Default {
              n78 = case shown="\"Frequency\", Default" w240 {
                tunnel: w239 -> [w249 w258 w267 w276]
                tunnel: w238 -> [w248 w257 w266 w275]
                tunnel: [w247 w256 w265 w274] -> w233
                tunnel: [REF_Parameter--Enum."Frequency" ("Parameter") REF_Parameter--Enum."Phase" ("Parameter") REF_Parameter--Enum."Time Constant" ("Parameter") REF_Parameter--Enum."RollOff" ("Parameter")] -> w234
                tunnel: [w245 w254 w263 w272] -> w231
                tunnel: [w243 w252 w261 w270] -> w232
                frame "Frequency", Default {
                  n79 = call "From JSON Text.vim"("Data Type and Default Value"=T19 {"Channel"=0, "Frequency"=0.0} ("setREF_f"), "error in (no error)"=w248, "JSON"=w249) -> ("error out"=w247:errorcluster, "Data out"=w246:T19)  [unwired: 7 in]
                  n80 = Unbundle By Name(w246) -> ("Channel"=w245:i32, "Frequency"=w244:dbl)
                  n81 = To Variant(anything=w244) -> (Variant=w243:variant)
                }
                frame "Phase" {
                  n82 = call "From JSON Text.vim"("Data Type and Default Value"=T21 {"Channel"=0, "Phase"=0.0} ("setREF_phi"), "error in (no error)"=w257, "JSON"=w258) -> ("error out"=w256:errorcluster, "Data out"=w255:T21)  [unwired: 7 in]
                  n83 = Unbundle By Name(w255) -> ("Channel"=w254:i32, "Phase"=w253:dbl)
                  n84 = To Variant(anything=w253) -> (Variant=w252:variant)
                }
                frame "TC" {
                  n85 = call "From JSON Text.vim"("Data Type and Default Value"=T22 {"Channel"=0, "TC"=1e-05} ("setREF_phi"), "error in (no error)"=w266, "JSON"=w267) -> ("error out"=w265:errorcluster, "Data out"=w264:T22)  [unwired: 7 in]
                  n86 = Unbundle By Name(w264) -> ("Channel"=w263:i32, "TC"=w262:dbl)
                  n87 = To Variant(anything=w262) -> (Variant=w261:variant)
                }
                frame "RollOff" {
                  n88 = call "From JSON Text.vim"("Data Type and Default Value"=T23 {"Channel"=0, "Roll-Off"=1} ("setREF_Roll-Off"), "error in (no error)"=w275, "JSON"=w276) -> ("error out"=w274:errorcluster, "Data out"=w273:T23)  [unwired: 7 in]
                  n89 = Unbundle By Name(w273) -> ("Channel"=w272:i32, "Roll-Off"=w271:i32)
                  n90 = To Variant(anything=w271) -> (Variant=w270:variant)
                }
              }
              n91 = call "Update REF Parameter.vi"("Parameter"=w234, "error in"=w233, "Value"=w232, "Channel"=w231, "Instrument.Lockin"=w237) -> ("error out"=w235:errorcluster, "Instrument.Lockin out"=w236:refnum<class "Instrument.Lockin.lvclass">)  [unwired: 5 in]
            }
            frame "" {
              n92 = call "From JSON Text.vim"("Data Type and Default Value"=T24 [] ("REF Channels"), "error in (no error)"=w282, "JSON"=w283) -> ("error out"=w278:errorcluster, "Data out"=w279:T24)  [unwired: 7 in]
              n93 = Bundle By Name(cluster=w281, "Cfg_REF"=w279) -> (w280:refnum<class "Instrument.Lockin.lvclass">)
            }
          }
          n94 = Unbundle By Name(w218) -> ("Instrument.DAQ"=w222:refnum<class "Instrument.DAQ.lvclass">, "Cfg_REF"=w216:T24)
          n95 = call "DAQ.setREF.vi"("error in (no error)"=w217, "Channels: Lockin"=w216, "Instrument.DAQ"=w222) -> ("error out"=w220:errorcluster, "Instrument.DAQ out"=w221:refnum<class "Instrument.DAQ.lvclass">)  [unwired: 7 in]
          n96 = disable-structure shown="Disabled" {
            disable-tunnel: w221 -> [w229 _]
            disable-tunnel: w220 -> [w228 w230]
            disable-tunnel: [w227 w230] -> w219
            frame Disabled {
              # "Lockin SMO: Reset Phase"
              n97 = call "DAQ.zeroPhase.vi"("error in (no error)"=w228, "Instrument.DAQ"=w229) -> ("error out"=w227:errorcluster)  [unwired: 8 in, 1 out]
            }
            frame Enabled {
            }
          }
        }
        frame "setSweep" {
          n98 = Unbundle By Name(w286) -> ("Sweep"=w285:T49)
          n99 = case shown="\"Time\"" w287 {
            tunnel: w294 -> [w298 w307 w314]
            tunnel: w293 -> [w297 w306 w313]
            tunnel: [w296 w305 w312] -> w292
            tunnel: [w295 w301 w310] -> w284
            tunnel: w285 -> [_ w303 w311]
            frame "", Default {
              w299 = T49 {"sweepTime"=0.0, "initialWaitTime"=0.0, "returnToStart"=FALSE, "sweepChannels"=[]}  # Configure Sweep
              n100 = call "From JSON Text.vim"("Data Type and Default Value"=w299, "error in (no error)"=w297, "JSON"=w298) -> ("error out"=w296:errorcluster, "Data out"=w295:T49)  [unwired: 7 in]
            }
            frame "Time" {
              n101 = call "From JSON Text.vim"("Data Type and Default Value"=T26 {"SweepTime"=0.0} ("setSweep_Time"), "error in (no error)"=w306, "JSON"=w307) -> ("error out"=w305:errorcluster, "Data out"=w302:T26)  [unwired: 7 in]
              n102 = Unbundle By Name(w302) -> ("SweepTime"=w300:dbl)
              n103 = Bundle By Name(cluster=w303, "sweepTime"=w300) -> (w301:T49)
            }
            frame "Table" {
              n104 = call "From JSON Text.vim"("Data Type and Default Value"=T27[] [] ("Array"), "error in (no error)"=w313, "JSON"=w314) -> ("error out"=w312:errorcluster, "Data out"=w308:T27[])  [unwired: 7 in]
              n105 = call "Replace Sweep Waveforms.vi"("Channels New"=w308, "Sweep in"=w311) -> ("Sweep out"=w310:T49)  [unwired: 9 in]
            }
          }
          n106 = Bundle By Name(cluster=w286, "Sweep"=w284) -> (w290:refnum<class "Instrument.Lockin.lvclass">)
          n107 = Unbundle By Name(w290) -> ("Instrument.DAQ"=w289:refnum<class "Instrument.DAQ.lvclass">, "Sweep"=w288:T49)
          n108 = call "DAQ.setSweep.vi"("error in (no error)"=w292, "setSweep"=w288, "Instrument.DAQ"=w289) -> ("error out"=w291:errorcluster)  [unwired: 7 in, 1 out]
        }
        frame "setSampling" {
          n109 = call "From JSON Text.vim"("Data Type and Default Value"=T28 {"Fs"=204789.0, "#s"=15753}, "error in (no error)"=w322, "JSON"=w324) -> ("error out"=w315:errorcluster, "Data out"=w316:T28)  [unwired: 7 in]
          n110 = Bundle By Name(cluster=w318, "Sampling"=w316) -> (w317:refnum<class "Instrument.Lockin.lvclass">)
          n111 = Unbundle By Name(w317) -> ("Instrument.DAQ"=w321:refnum<class "Instrument.DAQ.lvclass">, "Sampling"=w319:T53)
          n112 = call "DAQ.setSampling.vi"("error in (no error)"=w315, "Sampling"=w319, "Instrument.DAQ"=w321) -> ("error out"=w320:errorcluster)  [unwired: 7 in, 1 out]
        }
        frame "setInputGain" {
          n113 = call "From JSON Text.vim"("Data Type and Default Value"=dbl[] [], "error in (no error)"=w336, "JSON"=w337) -> ("error out"=w335:errorcluster, "Data out"=w328:dbl[])  [unwired: 7 in]
          n114 = for {
            tunnel: T29 {"Channel"="AI1", "Gain"=1.0} ("System Cluster") -> [w342]
            tunnel: w328 -> [w341] mode=indexing
            tunnel: [w340] -> w327 mode=indexing
            n115 = Bundle By Name(cluster=w342, "Gain"=w341) -> (w340:T29)
          }
          n116 = Bundle By Name(cluster=w331, "Gain_AI"=w327) -> (w332:refnum<class "Instrument.Lockin.lvclass">)
          n117 = Unbundle By Name(w332) -> ("Instrument.DAQ"=w334:refnum<class "Instrument.DAQ.lvclass">, "Gain_AI"=w326:T47)
          n118 = for {
            tunnel: w326 -> [w339] mode=indexing
            tunnel: [w338] -> w325 mode=indexing
            n119 = Unbundle By Name(w339) -> ("Gain"=w338:dbl)
          }
          n120 = call "DAQ.setInputGain.vi"("error in (no error)"=w335, "Input Gain"=w325, "Instrument.DAQ"=w334) -> ("error out"=w333:errorcluster)  [unwired: 7 in, 1 out]
        }
        frame "setOffset" {
          n121 = call "From JSON Text.vim"("Data Type and Default Value"=dbl[] [], "error in (no error)"=w354, "JSON"=w355) -> ("error out"=w353:errorcluster, "Data out"=w346:dbl[])  [unwired: 7 in]
          n122 = for {
            tunnel: T29 {"Channel"="AI1", "Gain"=1.0} ("System Cluster") -> [w360]
            tunnel: w346 -> [w359] mode=indexing
            tunnel: [w358] -> w345 mode=indexing
            n123 = Bundle By Name(cluster=w360, "Gain"=w359) -> (w358:T29)
          }
          n124 = Bundle By Name(cluster=w349, "Offset_AI"=w345) -> (w350:refnum<class "Instrument.Lockin.lvclass">)
          n125 = Unbundle By Name(w350) -> ("Instrument.DAQ"=w352:refnum<class "Instrument.DAQ.lvclass">, "Offset_AI"=w344:T47)
          n126 = for {
            tunnel: w344 -> [w357] mode=indexing
            tunnel: [w356] -> w343 mode=indexing
            n127 = Unbundle By Name(w357) -> ("Gain"=w356:dbl)
          }
          n128 = call "DAQ.setInputOffset.vi"("error in (no error)"=w353, "Input Offset"=w343, "Instrument.DAQ"=w352) -> ("error out"=w351:errorcluster)  [unwired: 7 in, 1 out]
        }
        frame "setOutputGain" {
          n129 = call "From JSON Text.vim"("Data Type and Default Value"=dbl[] [], "error in (no error)"=w372, "JSON"=w373) -> ("error out"=w367:errorcluster, "Data out"=w364:dbl[])  [unwired: 7 in]
          n130 = for {
            tunnel: T29 {"Channel"="AI1", "Gain"=1.0} ("System Cluster") -> [w378]
            tunnel: w364 -> [w377] mode=indexing
            tunnel: [w376] -> w363 mode=indexing
            n131 = Bundle By Name(cluster=w378, "Gain"=w377) -> (w376:T29)
          }
          n132 = Bundle By Name(cluster=w368, "Gain_AO"=w363) -> (w369:refnum<class "Instrument.Lockin.lvclass">)
          n133 = Unbundle By Name(w369) -> ("Instrument.DAQ"=w371:refnum<class "Instrument.DAQ.lvclass">, "Gain_AO"=w362:T47)
          n134 = for {
            tunnel: w362 -> [w375] mode=indexing
            tunnel: [w374] -> w361 mode=indexing
            n135 = Unbundle By Name(w375) -> ("Gain"=w374:dbl)
          }
          n136 = call "DAQ.setOutputGain.vi"("error in (no error)"=w367, "Output Gain"=w361, "Instrument.DAQ"=w371) -> ("error out"=w370:errorcluster)  [unwired: 7 in, 1 out]
        }
        frame "setDAQ" {
          n137 = call "From JSON Text.vim"("Data Type and Default Value"=T30 [] ("DAQ.Config []"), "error in (no error)"=w393, "JSON"=w394) -> ("error out"=w383:errorcluster, "Data out"=w391:T30)  [unwired: 7 in]
          n138 = call "config UI to not UI (AO and AI).vi"("New Ch []"=w391) -> ("AO Config"=w380:T54, "AI Config"=w379:T56)  [unwired: 9 in]
          n139 = Bundle By Name(cluster=w385, "AI"=w379, "AO"=w380) -> (w384:refnum<class "Instrument.Lockin.lvclass">)
          n140 = Unbundle By Name(w384) -> ("Instrument.DAQ"=w386:refnum<class "Instrument.DAQ.lvclass">, "AI"=w388:T56, "Simulation mode"=w381:T39, "AO"=w387:T54)
          n141 = call "DAQ.setAIconfig.vi"("error in (no error)"=w383, "Simulation mode"=w381, "AI Configuration"=w388, "Instrument.DAQ"=w386) -> ("error out"=w390:errorcluster, "Instrument.DAQ out"=w392:refnum<class "Instrument.DAQ.lvclass">)  [unwired: 6 in]
          n142 = call "DAQ.setAOconfig.vi"("error in (no error)"=w390, "AO Configuration"=w387, "Instrument.DAQ"=w392) -> ("error out"=w389:errorcluster)  [unwired: 7 in, 1 out]
        }
        frame "----------LOCAL API----------" {
        }
        frame "showUI" {
          n143 = call "From JSON Text.vim"("Data Type and Default Value"=T36 FALSE ("show UI?"), "error in (no error)"=w401, "JSON"=w404) -> ("error out"=w400:errorcluster, "Data out"=w402:T36)  [unwired: 7 in]
          n144 = Unbundle By Name(w398) -> ("Instrument.DAQ"=w397:refnum<class "Instrument.DAQ.lvclass">)
          n145 = call "DAQ.showUI.vi"("error in (no error)"=w400, "show UI?"=w402, "Instrument.DAQ"=w397) -> ("error out"=w399:errorcluster)  [unwired: 7 in, 1 out]
        }
        frame "setAI" {
          # "Lockin SMO: Set AI"
          n146 = call "From JSON Text.vim"("Data Type and Default Value"=T37 [] ("AI Channels"), "error in (no error)"=w413, "JSON"=w414) -> ("error out"=w407:errorcluster, "Data out"=w405:T37)  [unwired: 7 in]
          n147 = Bundle By Name(cluster=w412, "Cfg_AI"=w405) -> (w406:refnum<class "Instrument.Lockin.lvclass">)
          n148 = Unbundle By Name(w406) -> ("Instrument.DAQ"=w410:refnum<class "Instrument.DAQ.lvclass">, "Cfg_AI"=w409:T37)
          n149 = call "DAQ.setAI.vi"("error in (no error)"=w407, "AI Channels"=w409, "Instrument.DAQ"=w410) -> ("error out"=w408:errorcluster)  [unwired: 7 in, 1 out]
        }
        frame "setData" {
          n150 = case shown="\"OutputGain\"" w419 {
            tunnel: w420 -> [w422 w431 w442 w451 w453 w465 w477 w496 w505 w514 w523 w532]
            tunnel: w418 -> [_ w428 w437 w448 w456 w468 w479 w492 w502 w507 w520 w529]
            tunnel: w417 -> [w421 w424 w436 w447 w455 w467 w480 w491 w500 w511 w519 w528]
            tunnel: [w422 w430 w441 w450 w452 w464 w476 w495 w504 w513 w522 w531] -> w416
            tunnel: [w421 w426 w434 w445 w454 w466 w478 w489 w498 w509 w517 w526] -> w415
            frame Default {
            }
            frame "State" {
              n151 = Unbundle By Name(w431) -> ("DAQ State"=w423:T46)
              n152 = Unflatten From String(type=w423, binary string=w428, error in (no error)=w424) -> (value=w429:T46, error out=w427:errorcluster)  [unwired: 2 in, 1 out]
              n153 = Variant To Data(error in=w427, type=w423, Variant=w429) -> (data=w425:T46, error out=w426:errorcluster)
              n154 = Bundle By Name(cluster=w431, "DAQ State"=w425) -> (w430:refnum<class "Instrument.Lockin.lvclass">)
            }
            frame "DAQ" {
              w432 = T30 [] ("DAQ.Config []")
              # "only setData is flatten to string. otherwise use JSON"
              n155 = Unflatten From String(type=w432, binary string=w437, error in (no error)=w436) -> (value=w438:T30, error out=w435:errorcluster)  [unwired: 2 in, 1 out]
              n156 = Variant To Data(error in=w435, type=w432, Variant=w438) -> (data=w433:T30, error out=w434:errorcluster)
              n157 = call "config UI to not UI (AO and AI).vi"("New Ch []"=w433) -> ("AO Config"=w440:T54, "AI Config"=w439:T56)  [unwired: 9 in]
              n158 = Bundle By Name(cluster=w442, "AI"=w439, "AO"=w440) -> (w441:refnum<class "Instrument.Lockin.lvclass">)
            }
            frame "Sampling" {
              n159 = Unbundle By Name(w451) -> ("Sampling"=w443:T53)
              n160 = Unflatten From String(type=w443, binary string=w448, error in (no error)=w447) -> (value=w449:T53, error out=w446:errorcluster)  [unwired: 2 in, 1 out]
              n161 = Variant To Data(error in=w446, type=w443, Variant=w449) -> (data=w444:T53, error out=w445:errorcluster)
              n162 = Bundle By Name(cluster=w451, "Sampling"=w444) -> (w450:refnum<class "Instrument.Lockin.lvclass">)
            }
            frame "Waveforms" {
              n163 = in-place {
                in-place-border: w456 -> [w462]
                in-place-border: w455 -> [w461]
                in-place-border: [w459] -> w454
                n164 = in-place-cluster #1(w453) -> ("Waveforms"=w458:T57)
                n165 = Unflatten From String(type=w458, binary string=w462, error in (no error)=w461) -> (value=w463:T57, error out=w460:errorcluster)  [unwired: 2 in, 1 out]
                n166 = Variant To Data(error in=w460, type=w458, Variant=w463) -> (data=w457:T57, error out=w459:errorcluster)
                n167 = in-place-cluster #1("Waveforms"=w457) -> (w452:refnum<class "Instrument.Lockin.lvclass">)
              }
            }
            frame "Results" {
              n168 = in-place {
                in-place-border: w468 -> [w474]
                in-place-border: w467 -> [w473]
                in-place-border: [w471] -> w466
                n169 = in-place-cluster #2(w465) -> ("Results"=w469:T48)
                n170 = Unflatten From String(type=w469, binary string=w474, error in (no error)=w473) -> (value=w475:T48, error out=w472:errorcluster)  [unwired: 2 in, 1 out]
                n171 = Variant To Data(error in=w472, type=w469, Variant=w475) -> (data=w470:T48, error out=w471:errorcluster)
                n172 = in-place-cluster #2("Results"=w470) -> (w464:refnum<class "Instrument.Lockin.lvclass">)
              }
            }
            frame "SweepWaveforms" {
              n173 = in-place {
                in-place-border: w480 -> [w486]
                in-place-border: w479 -> [w485]
                in-place-border: [w483] -> w478
                n174 = in-place-cluster #3(w477) -> ("SweepWaveforms"=w482:T58)
                n175 = Unflatten From String(type=w482, binary string=w485, error in (no error)=w486) -> (value=w487:T58, error out=w484:errorcluster)  [unwired: 2 in, 1 out]
                n176 = Variant To Data(error in=w484, type=w482, Variant=w487) -> (data=w481:T58, error out=w483:errorcluster)
                n177 = in-place-cluster #3("SweepWaveforms"=w481) -> (w476:refnum<class "Instrument.Lockin.lvclass">)
              }
            }
            frame "AOChannels" {
              n178 = Unbundle By Name(w496) -> ("Cfg_AO"=w488:T17)
              n179 = Unflatten From String(type=w488, binary string=w492, error in (no error)=w491) -> (value=w494:T17, error out=w490:errorcluster)  [unwired: 2 in, 1 out]
              n180 = Variant To Data(error in=w490, type=w488, Variant=w494) -> (data=w493:T17, error out=w489:errorcluster)
              n181 = Bundle By Name(cluster=w496, "Cfg_AO"=w493) -> (w495:refnum<class "Instrument.Lockin.lvclass">)
            }
            frame "AIChannels" {
              n182 = Unbundle By Name(w505) -> ("Cfg_AI"=w497:T37)
              n183 = Unflatten From String(type=w497, binary string=w502, error in (no error)=w500) -> (value=w503:T37, error out=w499:errorcluster)  [unwired: 2 in, 1 out]
              n184 = Variant To Data(error in=w499, type=w497, Variant=w503) -> (data=w501:T37, error out=w498:errorcluster)
              n185 = Bundle By Name(cluster=w505, "Cfg_AI"=w501) -> (w504:refnum<class "Instrument.Lockin.lvclass">)
            }
            frame "REFChannels" {
              n186 = Unbundle By Name(w514) -> ("Cfg_REF"=w506:T24)
              n187 = Unflatten From String(type=w506, binary string=w507, error in (no error)=w511) -> (value=w512:T24, error out=w510:errorcluster)  [unwired: 2 in, 1 out]
              n188 = Variant To Data(error in=w510, type=w506, Variant=w512) -> (data=w508:T24, error out=w509:errorcluster)
              n189 = Bundle By Name(cluster=w514, "Cfg_REF"=w508) -> (w513:refnum<class "Instrument.Lockin.lvclass">)
            }
            frame "InputGain" {
              n190 = Unbundle By Name(w523) -> ("Gain_AI"=w515:T47)
              n191 = Unflatten From String(type=w515, binary string=w520, error in (no error)=w519) -> (value=w521:T47, error out=w518:errorcluster)  [unwired: 2 in, 1 out]
              n192 = Variant To Data(error in=w518, type=w515, Variant=w521) -> (data=w516:T47, error out=w517:errorcluster)
              n193 = Bundle By Name(cluster=w523, "Gain_AI"=w516) -> (w522:refnum<class "Instrument.Lockin.lvclass">)
            }
            frame "OutputGain" {
              n194 = Unbundle By Name(w532) -> ("Gain_AO"=w524:T47)
              n195 = Unflatten From String(type=w524, binary string=w529, error in (no error)=w528) -> (value=w530:T47, error out=w527:errorcluster)  [unwired: 2 in, 1 out]
              n196 = Variant To Data(error in=w527, type=w524, Variant=w530) -> (data=w525:T47, error out=w526:errorcluster)
              n197 = Bundle By Name(cluster=w532, "Gain_AO"=w525) -> (w531:refnum<class "Instrument.Lockin.lvclass">)
            }
          }
        }
        frame "autoConfigureDAQ" {
          n198 = Unbundle By Name(w534) -> ("Instrument.DAQ"=w533:refnum<class "Instrument.DAQ.lvclass">)
          n199 = call "DAQ.autoConfigureDAQ.vi"("error in (no error)"=w535, "Instrument.DAQ"=w533) -> ("error out"=w536:errorcluster)  [unwired: 8 in, 1 out]
        }
        frame "setSimulationMode" {
          n200 = call "From JSON Text.vim"("Data Type and Default Value"=Simulation_Mode--enum."AI = noise*AO" ("AI Simulation mode"), "error in (no error)"=w540, "JSON"=w541) -> ("error out"=w539:errorcluster, "Data out"=w537:T39)  [unwired: 7 in]
          n201 = Bundle By Name(cluster=w547, "Simulation mode"=w537) -> (w546:refnum<class "Instrument.Lockin.lvclass">)
          n202 = Unbundle By Name(w546) -> ("Instrument.DAQ"=w545:refnum<class "Instrument.DAQ.lvclass">, "AI"=w544:T56, "Simulation mode"=w543:T39)
          n203 = call "DAQ.setAIconfig.vi"("error in (no error)"=w539, "Simulation mode"=w543, "AI Configuration"=w544, "Instrument.DAQ"=w545) -> ("error out"=w542:errorcluster)  [unwired: 6 in, 1 out]
        }
        frame "setOffsetMode" {
          n204 = Build Array(Offset_Mode--Enum."Remove" ("Offset Mode")) -> (w549:T40[])
          n205 = call "From JSON Text.vim"("Data Type and Default Value"=w549, "error in (no error)"=w551, "JSON"=w554) -> ("error out"=w550:errorcluster, "Data out"=w552:T40[])  [unwired: 7 in]
          n206 = Index Array(array=w552) -> (element=w548:T40)  [unwired: 1 in]
          n207 = Unbundle By Name(w557) -> ("Instrument.DAQ"=w556:refnum<class "Instrument.DAQ.lvclass">)
          n208 = case shown="\"Measure\"" w548 {
            tunnel: w556 -> [w560 w563]
            tunnel: w550 -> [w559 w562]
            tunnel: [w558 w561] -> w555
            frame "Measure" {
              n209 = call "DAQ.measureOffset.vi"("error in (no error)"=w559, "Instrument.DAQ"=w560) -> ("error out"=w558:errorcluster)  [unwired: 8 in, 1 out]
            }
            frame "Remove" {
              n210 = call "DAQ.zeroOffset.vi"("error in (no error)"=w562, "Instrument.DAQ"=w563) -> ("error out"=w561:errorcluster)  [unwired: 8 in, 1 out]
            }
          }
        }
        frame "zeroPhase" {
          n211 = Unbundle By Name(w567) -> ("Instrument.DAQ"=w564:refnum<class "Instrument.DAQ.lvclass">)
          n212 = call "DAQ.zeroPhase.vi"("error in (no error)"=w566, "Instrument.DAQ"=w564) -> ("error out"=w565:errorcluster)  [unwired: 8 in, 1 out]
        }
        frame "setCalibration" {
          n213 = call "From JSON Text.vim"("Data Type and Default Value"=PrivateEvents--DAQ.setCalibration."Check" ("setCalibration"), "error in (no error)"=w568, "JSON"=w572) -> ("error out"=w569:errorcluster, "Data out"=w570:T41)  [unwired: 7 in]
          n214 = Unbundle By Name(w575) -> ("Instrument.DAQ"=w574:refnum<class "Instrument.DAQ.lvclass">)
          n215 = call "DAQ.setCalibration.vi"("error in (no error)"=w569, "setCalibration"=w570, "Instrument.DAQ"=w574) -> ("error out"=w573:errorcluster)  [unwired: 7 in, 1 out]
        }
        frame "setPreFilter" {
          n216 = call "From JSON Text.vim"("Data Type and Default Value"=T42 {"60 Hz"=FALSE, "Low Pass"=FALSE, "Low Pass Cutoff (Hz)"=0.0} ("PreFilter"), "error in (no error)"=w577, "JSON"=w579) -> ("error out"=w576:errorcluster, "Data out"=w578:T42)  [unwired: 7 in]
          n217 = Bundle By Name(cluster=w582, "Prefilter"=w578) -> (w583:refnum<class "Instrument.Lockin.lvclass">)
          n218 = Unbundle By Name(w583) -> ("Instrument.DAQ"=w585:refnum<class "Instrument.DAQ.lvclass">, "Prefilter"=w581:T42)
          n219 = call "DAQ.setPreFilter.vi"("error in (no error)"=w576, "PreFilter"=w581, "Instrument.DAQ"=w585) -> ("error out"=w584:errorcluster)  [unwired: 7 in, 1 out]
        }
        frame "setFrequencyLink" {
          n220 = call "From JSON Text.vim"("Data Type and Default Value"=T43 {"Link?"=FALSE, "Frequency (Hz)"=0.0} ("Link Frequencies"), "error in (no error)"=w588, "JSON"=w590) -> ("error out"=w587:errorcluster, "Data out"=w586:T43)  [unwired: 7 in]
          n221 = Bundle By Name(cluster=w594, "Link Frequencies"=w586) -> (w595:refnum<class "Instrument.Lockin.lvclass">)
          n222 = Unbundle By Name(w595) -> ("Instrument.DAQ"=w593:refnum<class "Instrument.DAQ.lvclass">, "Link Frequencies"=w592:T43)
          n223 = call "DAQ.setLinkFrequencies.vi"("error in (no error)"=w587, "Link Frequencies"=w592, "Instrument.DAQ"=w593) -> ("error out"=w591:errorcluster)  [unwired: 7 in, 1 out]
        }
        frame "setAmplitudeLimit" {
          w599 = T59 {"Limit (V)"=0.0}  # Limit Amplitude
          n224 = call "From JSON Text.vim"("Data Type and Default Value"=w599, "error in (no error)"=w597, "JSON"=w600) -> ("error out"=w596:errorcluster, "Data out"=w598:T59)  [unwired: 7 in]
          n225 = Bundle By Name(cluster=w604, "Amplitude Limit"=w598) -> (w605:refnum<class "Instrument.Lockin.lvclass">)
          n226 = Unbundle By Name(w605) -> ("Instrument.DAQ"=w603:refnum<class "Instrument.DAQ.lvclass">, "Amplitude Limit"=w602:T59)
          n227 = call "DAQ.setAmplitudeLimit.vi"("error in (no error)"=w596, "Amplitude Limit"=w602, "Instrument.DAQ"=w603) -> ("error out"=w601:errorcluster)  [unwired: 7 in, 1 out]
        }
        frame "setDCLimit" {
          n228 = call "From JSON Text.vim"("Data Type and Default Value"=T44 {"Limit (V)"=0.0} ("DC Limit"), "error in (no error)"=w611, "JSON"=w613) -> ("error out"=w608:errorcluster, "Data out"=w612:T44)  [unwired: 7 in]
          n229 = Bundle By Name(cluster=w614, "DC Limit"=w612) -> (w615:refnum<class "Instrument.Lockin.lvclass">)
          n230 = Unbundle By Name(w615) -> ("Instrument.DAQ"=w610:refnum<class "Instrument.DAQ.lvclass">, "DC Limit"=w609:T44)
          n231 = call "DAQ.setDCLimit.vi"("error in (no error)"=w608, "DC Limit"=w609, "Instrument.DAQ"=w610) -> ("error out"=w607:errorcluster)  [unwired: 7 in, 1 out]
        }
        frame "setDutyCycle" {
          n232 = call "From JSON Text.vim"("Data Type and Default Value"=T45 {"Option?"=FALSE, "Duty Cycle (%)"=0.0} ("Function Option"), "error in (no error)"=w621, "JSON"=w623) -> ("error out"=w617:errorcluster, "Data out"=w622:T45)  [unwired: 7 in]
          n233 = Bundle By Name(cluster=w624, "Duty Cycle"=w622) -> (w625:refnum<class "Instrument.Lockin.lvclass">)
          n234 = Unbundle By Name(w625) -> ("Instrument.DAQ"=w619:refnum<class "Instrument.DAQ.lvclass">, "Duty Cycle"=w618:T45)
          n235 = call "DAQ.setDutyCycle.vi"("error in (no error)"=w617, "Duty Cycle"=w618, "Instrument.DAQ"=w619) -> ("error out"=w616:errorcluster)  [unwired: 7 in, 1 out]
        }
        frame "setSamplingFsOutput" {
          n236 = call "From JSON Text.vim"("Data Type and Default Value"=0.0, "error in (no error)"=w628, "JSON"=w629) -> ("error out"=w627:errorcluster, "Data out"=w626:dbl)  [unwired: 7 in]
          n237 = Bundle By Name(cluster=w635, "Fs_Out"=w626) -> (w632:refnum<class "Instrument.Lockin.lvclass">)
          n238 = Unbundle By Name(w632) -> ("Instrument.DAQ"=w634:refnum<class "Instrument.DAQ.lvclass">, "Sampling"=w633:T53)
          n239 = call "DAQ.setSampling.vi"("error in (no error)"=w627, "Sampling"=w633, "Instrument.DAQ"=w634) -> ("error out"=w631:errorcluster)  [unwired: 7 in, 1 out]
        }
      }
    }
    frame Error {
    }
  }
  "error out" <- w7
  "Instrument.Lockin out" <- w6
  "Command" <- w3
  "Processed Data" <- w5
